vi "TDMS Timestamp and Data.vi"   [LabVIEW 2015]
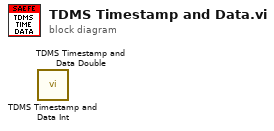
[diagram p0: block diagram]
diagram:
  n1 = call "TDMS Timestamp and Data Int.vi"() -> ()  [unwired: 10 in, 2 out]
  n2 = call "TDMS Timestamp and Data Double.vi"() -> ()  [unwired: 10 in, 2 out]
